vi "Error Code Window.vi"(7 "mode":T3 items=["create", "edit"], 8 "error in (no error)":errorcluster, 9 "selected error index":T2, 10 "scope":T1=enum."global", 11 "error list <top> in":variant) -> (0 "error out":errorcluster, 2 "modified?":bool, 3 "error list <top> out":variant)   [LabVIEW 2017]
uses:
  Controls/Error Code Window Modes.ctl
  Error List/Error Owner and ID.ctl
  Error List/Scope.ctl
  Controls/Error Code Window Data.ctl
  Controls/Error Code Window States.ctl
  <vilib>/Utility/miscctls.llb/LVPointTypeDef.ctl
  Error File Management/Controls/NI Error.ctl
  Error File Management/Error File Management.lvlib
panel:
  out "frame name (create)":string="New Error Code"
  out "frame name (edit)":string="Error Code"
  out "existing owner":string
  in  "owner":u16(ring) caption="Owner File"
  in  "error?":bool=TRUE
  in  "explore":bool
  in  "cancel":bool
  in  "ok":bool
  in  "code":i32 caption="Code"
  out "warning":bool
  in  "description":string caption="Description (Optional)"
  in  "remove":bool
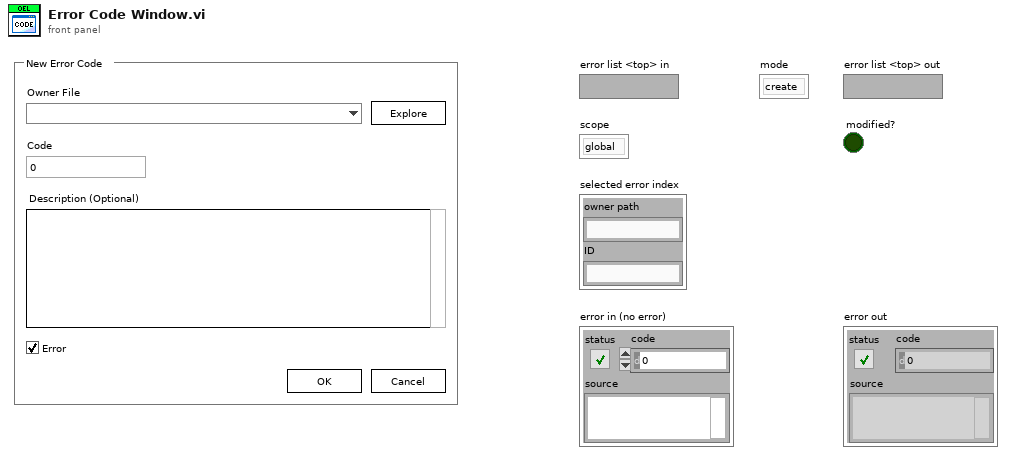
[diagram p1: front panel]
types:
  T1 = typedef "Scope.ctl" = enum16{"project", "global"}
  T2 = typedef "Error Owner and ID.ctl" = cluster{"owner path":string, "ID":string}
  T3 = typedef "Error Code Window Modes.ctl" = u8
  T4 = typedef "Error Code Window States.ctl" = enum16{"init", "load", "open FP", "idle", "modify", "close"}
  T5 = typedef "Error Code Window Data.ctl" = cluster{"state":T4, "mode":T3, "selected error ID":T2, "selected error code":i32, "owner path":path, "error codes":i32[], "existing error ID":T2, "exist?":bool, "modified?":bool, "error list <top>":variant, "scope":T1, "parsable error files":path[], "error files":path[], "error attributes":string[]}
  T6 = typedef "LVPointTypeDef.ctl" = cluster{"Horizontal":i16, "Vertical":i16}
  T7 = enum8{"Enabled", "Disabled", "Disabled and Grayed Out"}
  T8 = typedef "Error File Management.lvlib/NI Error.ctl" = errorcluster
  T9 = typedef "Error Code File Properties.ctl" = cluster{"path":path, "simplified path":string, "name":string, "display name":string, "family name":string, "comment":string, "parsable?":bool, "file modified?":bool}
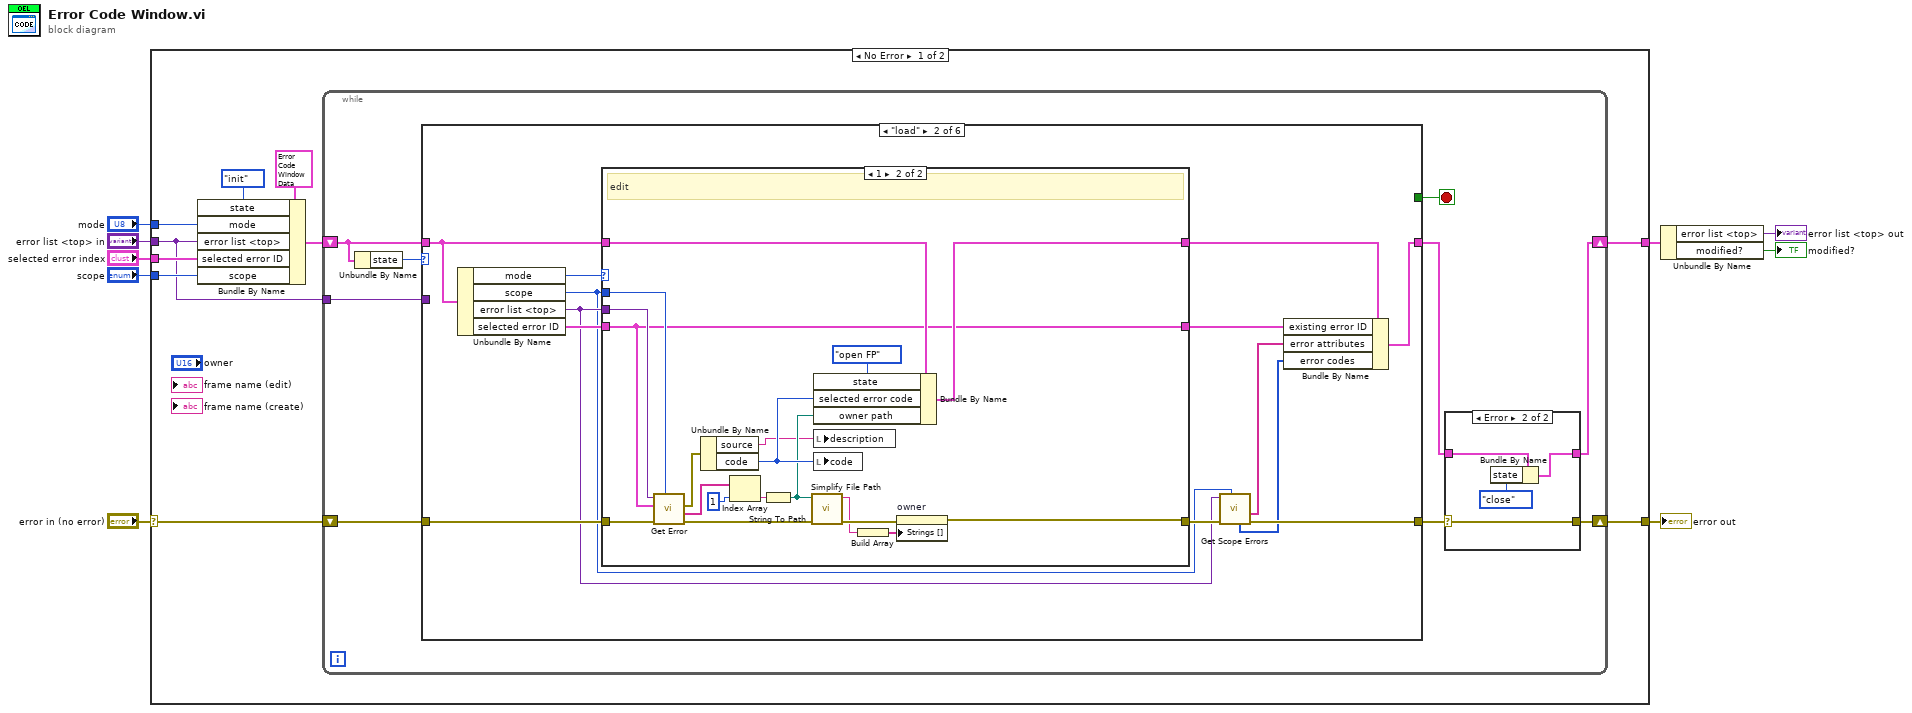
[diagram p0: block diagram]
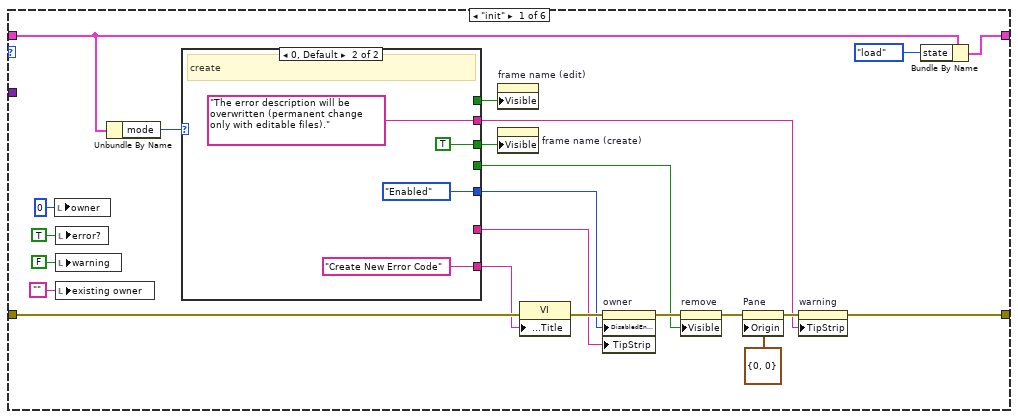
[diagram p2: hidden frame]
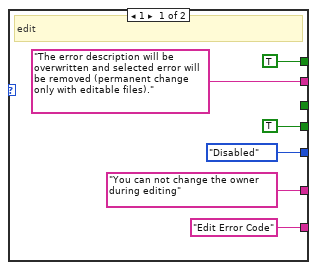
[diagram p3: hidden frame]
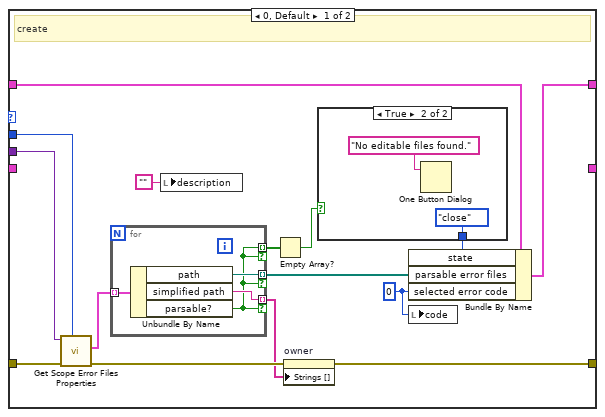
[diagram p4: hidden frame]
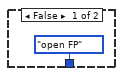
[diagram p5: hidden frame]
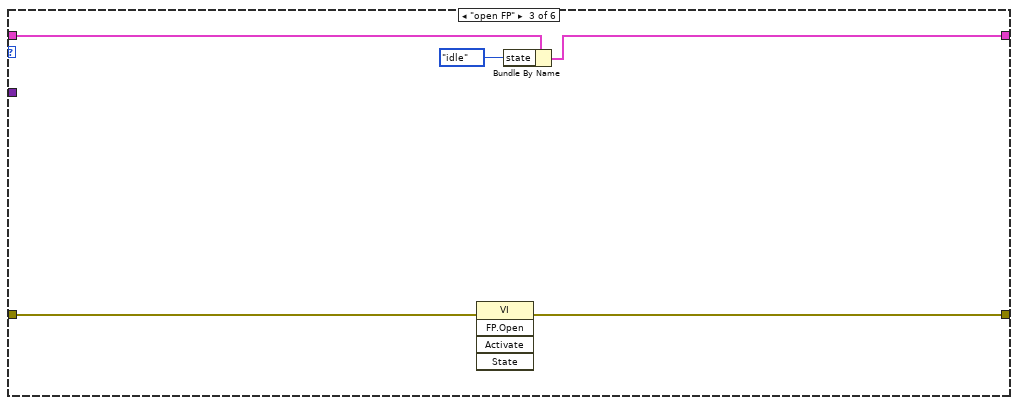
[diagram p6: hidden frame]
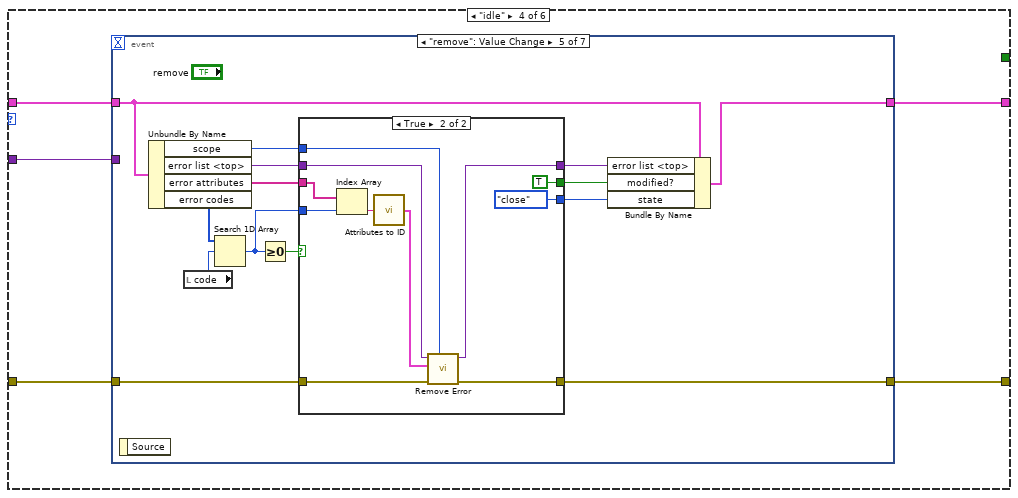
[diagram p7: hidden frame]
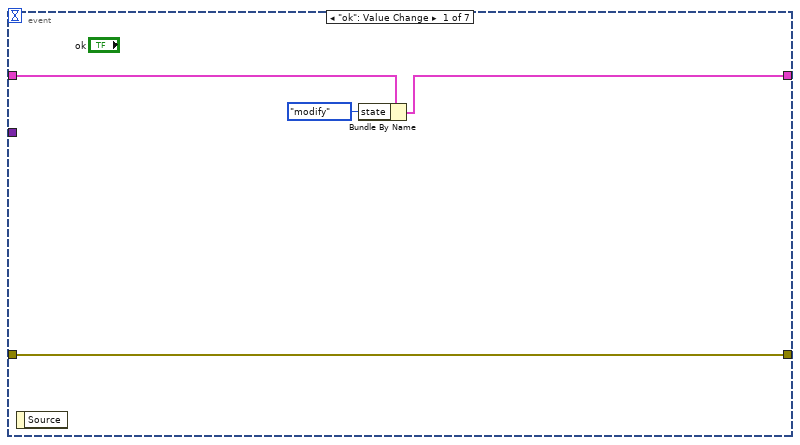
[diagram p8: hidden frame]
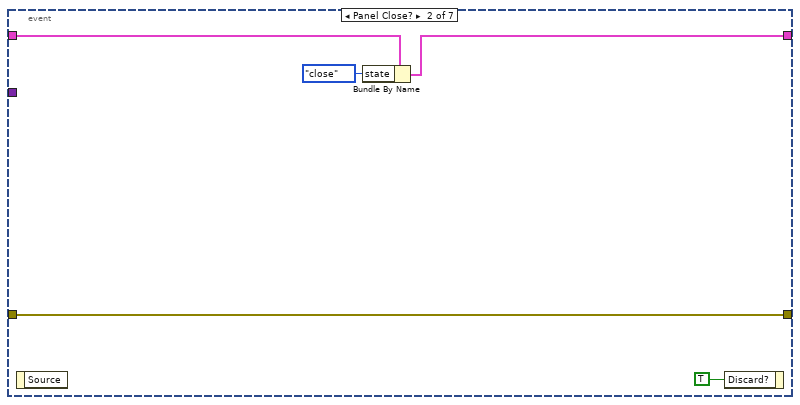
[diagram p9: hidden frame]
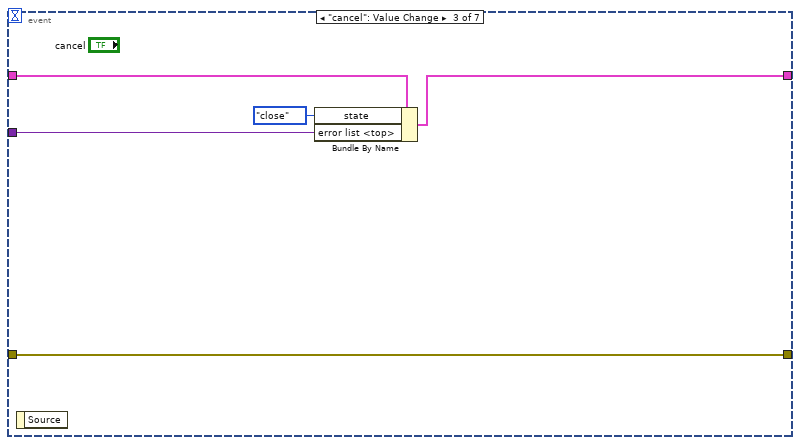
[diagram p10: hidden frame]
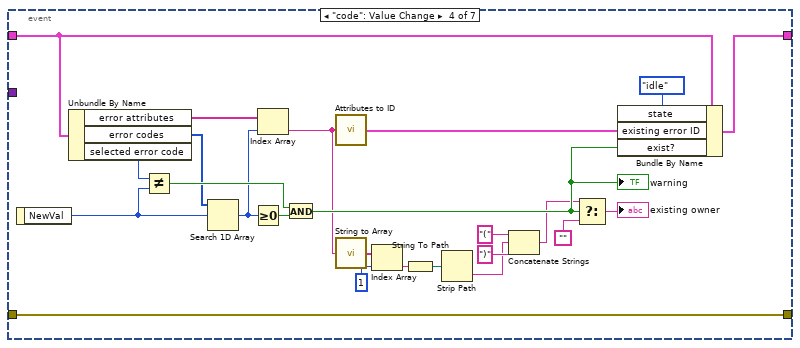
[diagram p11: hidden frame]
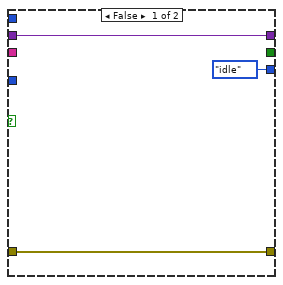
[diagram p12: hidden frame]
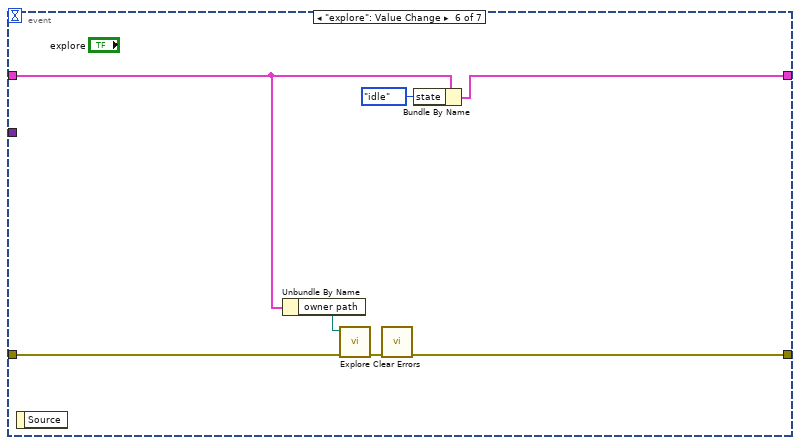
[diagram p13: hidden frame]
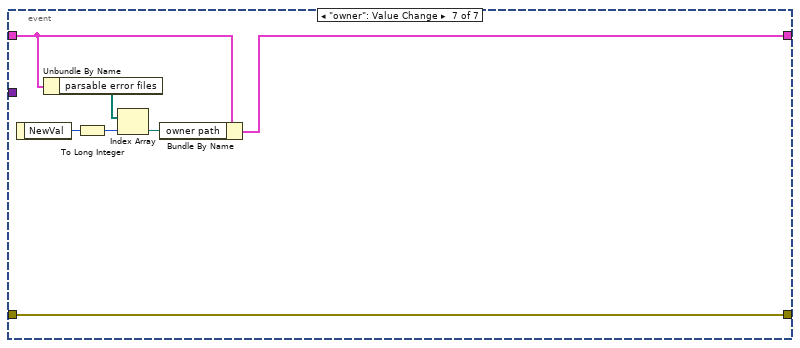
[diagram p14: hidden frame]
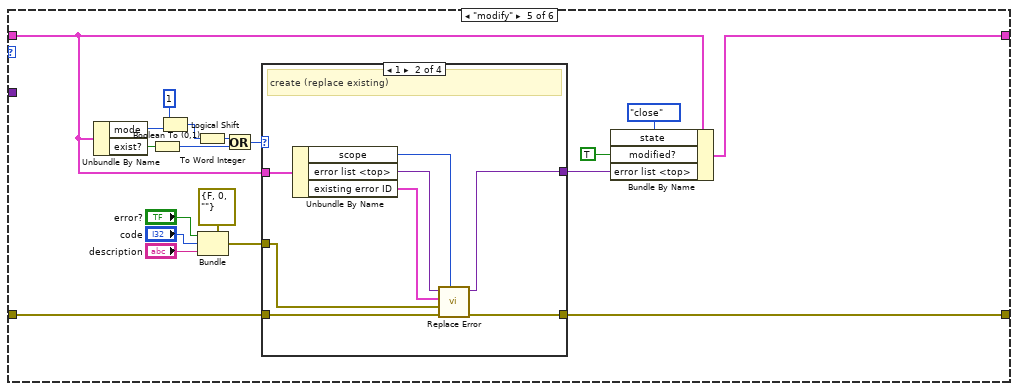
[diagram p15: hidden frame]
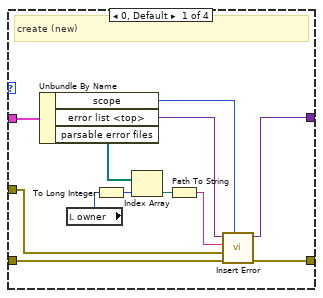
[diagram p16: hidden frame]
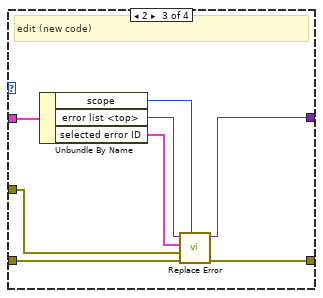
[diagram p17: hidden frame]
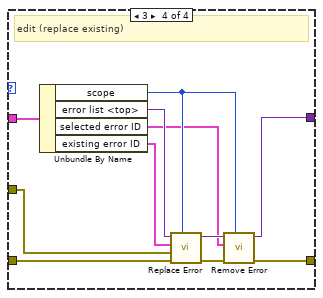
[diagram p18: hidden frame]
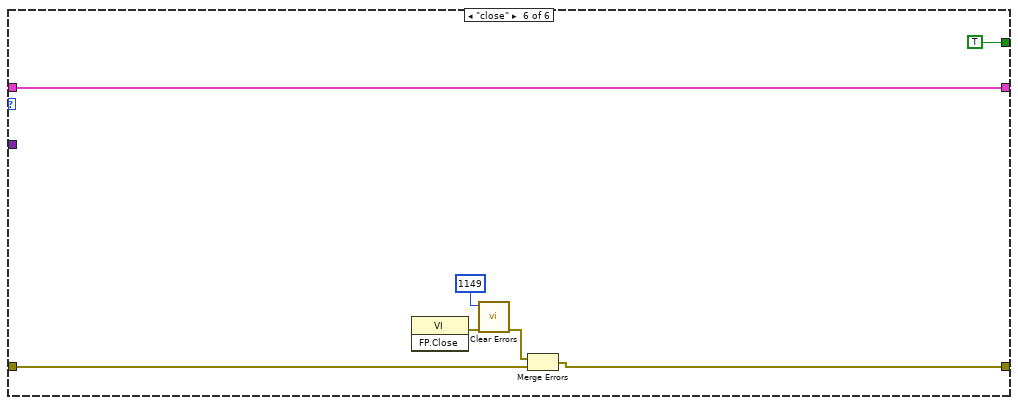
[diagram p19: hidden frame]
diagram:
  n1 = case shown="No Error" "error in (no error)" {
    selector: "error in (no error)" -> [w13 w276]
    tunnel: "selected error index" -> [w18 _]
    tunnel: "mode" -> [w19 _]
    tunnel: [w17 _] -> w6
    tunnel: "error list <top> in" -> [w10 _]
    tunnel: [w12 w276] -> w3
    tunnel: "scope" -> [w11 _]
    frame No Error {
      n2 = Bundle By Name(cluster=T5 {"state"=enum."init", "mode"=1, "selected error ID"={"owner path"="", "ID"=""}, "selected error code"=0, "owner path"=path "", "error codes"=[], "existing error ID"={"owner path"="", "ID"=""}, "exist?"=FALSE, "modified?"=FALSE, "error list <top>"=variant(cluster{"path":path, "simplified path":string, "name":string, "display name":string, "family name":string, "comment":string, "parsable?":bool, "file modified?":bool}[] []), "scope"=enum."project", "parsable error files"=[], "error files"=[], "error attributes"=[]} ("output cluster"), "state"=Error_Code_Window_States."init", "mode"=w19, "error list <top>"=w10, "selected error ID"=w18, "scope"=w11) -> (w15:T5)
      n3 = while {
        shift-right: [w20] -> w17
        shift-left: w15 -> [w27]
        shift-right: [w22] -> w12
        shift-left: w13 -> [w25]
        tunnel: w10 -> [w24]
        stop <- w28 stop-if-true
        n4 = Unbundle By Name(w27) -> ("state"=w26:T4)
        n5 = case shown="\"load\"" w26 {
          tunnel: [_ _ _ _ _ TRUE] -> w28
          tunnel: w27 -> [w47 w70 w117 w124 w222 w269]
          tunnel: [w46 w61 w116 w123 w223 w269] -> w21
          tunnel: w25 -> [w49 w71 w119 w122 w221 w264]
          tunnel: [w33 w68 w118 w121 w220 w263] -> w23
          tunnel: w24 -> [_ _ _ w120 _ _]
          frame "init" {
            n6 = local write "owner"(u16 0) -> ()
            n7 = local write "error?"(TRUE ("error?")) -> ()
            n8 = local write "warning"(FALSE ("warning")) -> ()
            n9 = local write "existing owner"("") -> ()
            n10 = Unbundle By Name(w47) -> ("mode"=w45:T3)
            n11 = case shown="0, Default" w45 {
              tunnel: ["Edit Error Code" "Create New Error Code"] -> w48
              tunnel: [TRUE _] -> w39
              tunnel: [T7."Disabled" ("Disabled") T7."Enabled" ("Disabled")] -> w36
              tunnel: ["You can not change the owner during editing" ("Tip Strip") _] -> w35
              tunnel: [TRUE _] -> w31
              tunnel: [_ TRUE] -> w30
              tunnel: ["The error description will be overwritten and selected error will be removed (permanent change only with editable files)." ("Tip Strip") "The error description will be overwritten (permanent change only with editable files)." ("Tip Strip")] -> w29
              frame 1 {
                # "edit"
              }
              frame 0, Default {
                # "create"
              }
            }
            n12 = property on="frame name (edit)" class="Str"("Visible"=w31) -> ()  [unwired: 2 in, 2 out]
            n13 = property on="frame name (create)" class="Str"("Visible"=w30) -> ()  [unwired: 2 in, 2 out]
            n14 = property class="VI"(error in=w49, "Front Panel.Title"=w48) -> (error out=w37:errorcluster)  [unwired: 1 in, 1 out]
            n15 = property on="owner" class="Ring (strict)"(error in=w37, "DisabledEnum"=w36, "TipStrip"=w35) -> (error out=w50:errorcluster)  [unwired: 1 in, 1 out]
            n16 = property on="remove" class="Bool"(error in=w50, "Visible"=w39) -> (error out=w40:errorcluster)  [unwired: 1 in, 1 out]
            n17 = property on="Pane" class="Pane"(error in=w40, "Origin"=T6 {"Horizontal"=0, "Vertical"=0}) -> (error out=w34:errorcluster)  [unwired: 1 in, 1 out]
            n18 = property on="warning" class="Bool (strict)"(error in=w34, "TipStrip"=w29) -> (error out=w33:errorcluster)  [unwired: 1 in, 1 out]
            n19 = Bundle By Name(cluster=w47, "state"=Error_Code_Window_States."load") -> (w46:T5)
          }
          frame "load" {
            n20 = Unbundle By Name(w70) -> ("mode"=w73:T3, "scope"=w66:T1, "error list <top>"=w67:variant, "selected error ID"=w72:T2)
            n21 = case shown="1" w73 {
              tunnel: w72 -> [_ w104]
              tunnel: w67 -> [w81 w110]
              tunnel: w66 -> [w80 w109]
              tunnel: w71 -> [w79 w114]
              tunnel: [w85 w102] -> w69
              tunnel: w70 -> [w87 w113]
              tunnel: [w82 w112] -> w62
              tunnel: [_ w104] -> w65
              frame 0, Default {
                w84 = 0 ("code")
                # "create"
                n22 = call "Get Scope Error Files Properties.vi"("scope"=w80, "error in (no error)"=w79, "error list <top>"=w81) -> ("error out"=w78:errorcluster, "properties"=w77:T9[])  [unwired: 4 in, 3 out]
                n23 = for {
                  tunnel: w77 -> [w92] mode=indexing
                  tunnel: [w91] -> w74 mode=indexing if=w89
                  tunnel: [w90] -> w75 mode=indexing if=w89
                  tunnel: [w89] -> w76 mode=indexing if=w89
                  n24 = Unbundle By Name(w92) -> ("path"=w91:path, "simplified path"=w90:string, "parsable?"=w89:bool)
                }
                n25 = local write "description"("") -> ()
                n26 = Empty Array?(array=w76) -> (empty?=w86:bool)
                n27 = property on="owner" class="Ring (strict)"(error in=w78, "Strings []"=w75) -> (error out=w85:errorcluster)  [unwired: 1 in, 1 out]
                n28 = case shown="True" w86 {
                  tunnel: [Error_Code_Window_States."open FP" ("state") Error_Code_Window_States."close" ("state")] -> w83
                  frame False {
                  }
                  frame True {
                    n29 = One Button Dialog(message="No editable files found.") -> ()  [unwired: 1 in, 1 out]
                  }
                }
                n30 = Bundle By Name(cluster=w87, "state"=w83, "parsable error files"=w74, "selected error code"=w84) -> (w82:T5)
                n31 = local write "code"(w84) -> ()
              }
              frame 1 {
                # "edit"
                n32 = call "Get Error.vi"("scope"=w109, "error in (no error)"=w114, "owner error"=w104, "error list <top>"=w110) -> ("error out"=w99:errorcluster, "attributes"=w97:string[], "error"=w96:T8)  [unwired: 3 in, 2 out]
                n33 = Unbundle By Name(w96) -> ("source"=w98:string, "code"=w108:i32)
                n34 = Index Array(array=w97, index=1) -> (element=w107:string)
                n35 = String To Path(string=w107) -> (path=w106:path)
                n36 = call "Simplify File Path.vi"("error in (no error)"=w99, "full path"=w106) -> ("error out"=w103:errorcluster, "simplified path"=w101:string)  [unwired: 8 in]
                n37 = Bundle By Name(cluster=w113, "state"=Error_Code_Window_States."open FP", "selected error code"=w108, "owner path"=w106) -> (w112:T5)
                n38 = local write "description"(w98) -> ()
                n39 = local write "code"(w108) -> ()
                n40 = Build Array(w101) -> (w100:string[])
                n41 = property on="owner" class="Ring (strict)"(error in=w103, "Strings []"=w100) -> (error out=w102:errorcluster)  [unwired: 1 in, 1 out]
              }
            }
            n42 = call "Get Scope Errors.vi"("scope"=w66, "error in (no error)"=w69, "error list <top> in"=w67) -> ("error out"=w68:errorcluster, "attributes"=w64:string[], "error codes"=w63:i32[])  [unwired: 4 in, 2 out]
            n43 = Bundle By Name(cluster=w62, "existing error ID"=w65, "error attributes"=w64, "error codes"=w63) -> (w61:T5)
          }
          frame "open FP" {
            n44 = invoke class="VI" method="FP.Open"(error in=w119) -> (error out=w118:errorcluster)  [unwired: 4 in, 4 out]
            n45 = Bundle By Name(cluster=w117, "state"=Error_Code_Window_States."idle") -> (w116:T5)
          }
          frame "idle" {
            n46 = event shown="[4] \"remove\": Value Change" {
              selector: _ -> [_ _ _ _ _ _ _]
              dyn-events: _ -> [_ _ _ _ _ _ _]
              timeout: _ -> [_ _ _ _ _ _ _]
              tunnel: w124 -> [w127 w131 w137 w160 w176 w194 w201]
              tunnel: [w126 w130 w136 w159 w175 w193 w200] -> w123
              tunnel: w122 -> [w125 w129 w135 w145 w164 w192 w204]
              tunnel: [w125 w129 w135 w145 w163 w191 w204] -> w121
              tunnel: w120 -> [_ _ w134 _ _ _ _]
              event "ok": Value Change {
                n47 = event-data() -> ()  [unwired: 1 in, 1 out]
                n48 = Bundle By Name(cluster=w127, "state"=Error_Code_Window_States."modify") -> (w126:T5)
              }
              event Panel Close? {
                n49 = event-data() -> ()  [unwired: 1 in, 1 out]
                n50 = Bundle By Name(cluster=w131, "state"=Error_Code_Window_States."close") -> (w130:T5)
                n51 = event-data("Discard?"=TRUE) -> ()  [unwired: 1 in, 1 out]
              }
              event "cancel": Value Change {
                n52 = event-data() -> ()  [unwired: 1 in, 1 out]
                n53 = Bundle By Name(cluster=w137, "state"=Error_Code_Window_States."close", "error list <top>"=w134) -> (w136:T5)
              }
              event "code": Value Change {
                n54 = event-data() -> ("NewVal"=w157:i32)  [unwired: 1 in]
                n55 = Unbundle By Name(w160) -> ("error attributes"=w153:string[], "error codes"=w161:i32[], "selected error code"=w156:i32)
                n56 = Not Equal?(x=w156, y=w157) -> (x != y?=w162:bool)
                n57 = Search 1D Array(1D array=w161, element=w157) -> (index of element=w154:i32)  [unwired: 1 in]
                n58 = Greater Or Equal To 0?(x=w154) -> (x >= 0?=w155:bool)
                n59 = Index Array(array=w153, index=w154) -> (element=w144:string)
                n60 = And(x=w162, y=w155) -> (x .and. y?=w149:bool)
                "warning" <- w149
                n61 = call "Attributes to ID.vi"("attributes"=w144) -> ("owner and ID"=w152:T2)
                n62 = call "String to Array.vi"("string"=w144) -> ("array"=w143:string[])  [unwired: 1 in]
                n63 = Index Array(array=w143, index=1) -> (element=w142:string)
                n64 = String To Path(string=w142) -> (path=w140:path)
                n65 = Strip Path(path=w140) -> (name=w139:string)  [unwired: 1 out]
                n66 = Concatenate Strings("(" ("string"), w139, ")" ("string")) -> (w148:string)
                n67 = Select(t=w148, s=w149, f="") -> (s? t:f=→"existing owner":string)
                n68 = Bundle By Name(cluster=w160, "state"=Error_Code_Window_States."idle", "existing error ID"=w152, "exist?"=w149) -> (w159:T5)
              }
              event "remove": Value Change {
                n69 = event-data() -> ()  [unwired: 1 in, 1 out]
                n70 = Unbundle By Name(w176) -> ("scope"=w168:T1, "error list <top>"=w174:variant, "error attributes"=w169:string[], "error codes"=w171:i32[])
                n71 = local read "code"() -> (w170:i32)
                n72 = Search 1D Array(1D array=w171, element=w170) -> (index of element=w172:i32)  [unwired: 1 in]
                n73 = Greater Or Equal To 0?(x=w172) -> (x >= 0?=w167:bool)
                n74 = case shown="True" w167 {
                  tunnel: w174 -> [w179 w190]
                  tunnel: [w179 w189] -> w173
                  tunnel: w172 -> [_ w188]
                  tunnel: w169 -> [_ w187]
                  tunnel: w168 -> [_ w186]
                  tunnel: [Error_Code_Window_States."idle" ("state") Error_Code_Window_States."close" ("state")] -> w166
                  tunnel: [_ TRUE] -> w165
                  tunnel: w164 -> [w178 w181]
                  tunnel: [w178 w180] -> w163
                  frame False {
                  }
                  frame True {
                    n75 = Index Array(array=w187, index=w188) -> (element=w183:string)
                    n76 = call "Attributes to ID.vi"("attributes"=w183) -> ("owner and ID"=w182:T2)
                    n77 = call "Remove Error.vi"("scope"=w186, "error in (no error)"=w181, "selected error"=w182, "error list <top> in"=w190) -> ("error out"=w180:errorcluster, "error list <top> out"=w189:variant)  [unwired: 6 in]
                  }
                }
                n78 = Bundle By Name(cluster=w176, "error list <top>"=w173, "modified?"=w165, "state"=w166) -> (w175:T5)
              }
              event "explore": Value Change {
                n79 = event-data() -> ()  [unwired: 1 in, 1 out]
                n80 = Unbundle By Name(w194) -> ("owner path"=w197:path)
                n81 = call "Explore.vi"("error in (no error)"=w192, "file path"=w197) -> ("error out"=w196:errorcluster)  [unwired: 9 in]
                n82 = call <vilib>:"Clear Errors.vi"("error in (no error)"=w196) -> ("error out"=w191:errorcluster)  [unwired: 5 in, 1 out]
                n83 = Bundle By Name(cluster=w194, "state"=Error_Code_Window_States."idle") -> (w193:T5)
              }
              event "owner": Value Change {
                n84 = event-data() -> ("NewVal"=w202:u16)  [unwired: 1 in]
                n85 = Unbundle By Name(w201) -> ("parsable error files"=w203:path[])
                n86 = To Long Integer(number=w202) -> (32bit integer=w198:i32)
                n87 = Index Array(array=w203, index=w198) -> (element=w199:path)
                n88 = Bundle By Name(cluster=w201, "owner path"=w199) -> (w200:T5)
              }
            }
          }
          frame "modify" {
            n89 = Unbundle By Name(w222) -> ("mode"=w216:T3, "exist?"=w217:bool)
            n90 = Boolean To (0,1)(Boolean=w217) -> (0, 1=w213:i16)
            n91 = Logical Shift(y=i16 1, x=w216) -> (x << y=w214:T3)
            n92 = To Word Integer(number=w214) -> (16bit integer=w205:i16)
            n93 = Bundle(cluster=T8 {"status"=FALSE, "code"=0, "source"=""} ("error cluster"), "status"="error?", "code"="code", "source"="description") -> (w206:T8)
            n94 = Or(x=w205, y=w213) -> (x .or. y?=w212:i16)
            n95 = case shown="1" w212 {
              tunnel: [w230 w241 w249 w260] -> w211
              tunnel: w222 -> [w235 w243 w251 w262]
              tunnel: w221 -> [w233 w240 w247 w257]
              tunnel: [w232 w238 w246 w258] -> w220
              tunnel: w206 -> [w234 w239 w248 w256]
              frame 0, Default {
                # "create (new)"
                n96 = Unbundle By Name(w235) -> ("scope"=w229:T1, "error list <top>"=w231:variant, "parsable error files"=w228:path[])
                n97 = local read "owner"() -> (w227:u16)
                n98 = To Long Integer(number=w227) -> (32bit integer=w224:i32)
                n99 = Index Array(array=w228, index=w224) -> (element=w226:path)
                n100 = Path To String(path=w226) -> (string=w225:string)
                n101 = call "Insert Error.vi"("scope"=w229, "error in (no error)"=w233, "new error"=w234, "owner path"=w225, "error list <top> in"=w231) -> ("error out"=w232:errorcluster, "error list <top> out"=w230:variant)  [unwired: 5 in]
              }
              frame 1 {
                # "create (replace existing)"
                n102 = Unbundle By Name(w243) -> ("scope"=w237:T1, "error list <top>"=w242:variant, "existing error ID"=w236:T2)
                n103 = call "Replace Error.vi"("scope"=w237, "error in (no error)"=w240, "new error"=w239, "error owner and ID"=w236, "error list <top> in"=w242) -> ("error out"=w238:errorcluster, "error list <top> out"=w241:variant)  [unwired: 5 in]
              }
              frame 2 {
                # "edit (new code)"
                n104 = Unbundle By Name(w251) -> ("scope"=w245:T1, "error list <top>"=w250:variant, "selected error ID"=w244:T2)
                n105 = call "Replace Error.vi"("scope"=w245, "error in (no error)"=w247, "new error"=w248, "error owner and ID"=w244, "error list <top> in"=w250) -> ("error out"=w246:errorcluster, "error list <top> out"=w249:variant)  [unwired: 5 in]
              }
              frame 3 {
                # "edit (replace existing)"
                n106 = Unbundle By Name(w262) -> ("scope"=w254:T1, "error list <top>"=w261:variant, "selected error ID"=w253:T2, "existing error ID"=w252:T2)
                n107 = call "Replace Error.vi"("scope"=w254, "error in (no error)"=w257, "new error"=w256, "error owner and ID"=w252, "error list <top> in"=w261) -> ("error out"=w259:errorcluster, "error list <top> out"=w255:variant)  [unwired: 5 in]
                n108 = call "Remove Error.vi"("scope"=w254, "error in (no error)"=w259, "selected error"=w253, "error list <top> in"=w255) -> ("error out"=w258:errorcluster, "error list <top> out"=w260:variant)  [unwired: 6 in]
              }
            }
            n109 = Bundle By Name(cluster=w222, "state"=Error_Code_Window_States."close", "modified?"=TRUE, "error list <top>"=w211) -> (w223:T5)
          }
          frame "close" {
            n110 = invoke class="VI" method="FP.Close"() -> (error out=w267:errorcluster)  [unwired: 3 in, 2 out]
            n111 = call <vilib>:"Clear Errors.vi"("error in (no error)"=w267, "specific error code to clear (0: all)"=1149) -> ("error out"=w266:errorcluster)  [unwired: 4 in, 1 out]
            n112 = Merge Errors(w266, w264) -> (w263:errorcluster)
          }
        }
        n113 = case shown="Error" w23 {
          selector: w23 -> [w271 w273]
          tunnel: [w271 w273] -> w22
          tunnel: w21 -> [w270 w275]
          tunnel: [w270 w274] -> w20
          frame No Error {
          }
          frame Error {
            n114 = Bundle By Name(cluster=w275, "state"=Error_Code_Window_States."close") -> (w274:T5)
          }
        }
      }
    }
    frame Error {
    }
  }
  "error out" <- w3
  n115 = Unbundle By Name(w6) -> ("error list <top>"=→"error list <top> out":variant, "modified?"=→"modified?":bool)
